vi "Start Counter.vi"(8 "error in (no error)":errorcluster, 10 "ligne index":i32, 11 "Hardware Resources in":T1={"AI"={"task name"="", "task_ref"="", "physical channels"="Dev1/ai0:7", "channels config"={"input terminal configuration"=0, "minimum value"=-5.0, "maximum value"=5.0}, "rate"=1000.0}, "conversions"={"ai0"={"a"=0.0, "b"=0.0}, "ai1"={"a"=0.0, "b"=0.0}, "ai2"={"a"=0.0, "b"=0.0}, "ai3"={"a"=0.0, "b"=0.0}, "ai4"={"a"=0.0, "b"=0.0}}, "compteur 0"={"task name"="CTR", "task_ref"="", "ctr"="Dev1/ctr0:3", "coeff"=4000.0}, "compteur 1"={"task name"="CTR1", "task_ref"="", "ctr"="Dev1/ctr1", "coeff"=4000.0}, "compteur 2"={"task name"="CTR2", "task_ref"="", "ctr"="Dev1/ctr2", "coeff"=4000.0}, "compteur 3"={"task name"="CTR3", "task_ref"="", "ctr"="Dev1/ctr3", "coeff"=4000.0}} {"compteur 3"."coeff" format="%0.2f"; "compteur 2"."coeff" format="%0.2f"; "compteur 1"."coeff" format="%0.2f"; "compteur 0"."coeff" format="%0.2f"; "AI"."rate" format="%0.2f"; "AI"."channels config"."input terminal configuration" items=["Default"=-1, "RSE"=10083, "NRSE"=10078, "Differential"=10106, "Pseudodifferential"=12529]}) -> (0 "error out":errorcluster)   [LabVIEW 2014, in "PLS Acquisition.lvlib"]
doc: "Stops the acquisition."
uses:
  PLS Acquisition.lvlib
  Hardware Configuration.ctl
  Settings/conversion.ctl
  Settings/PLS Settings.lvlib
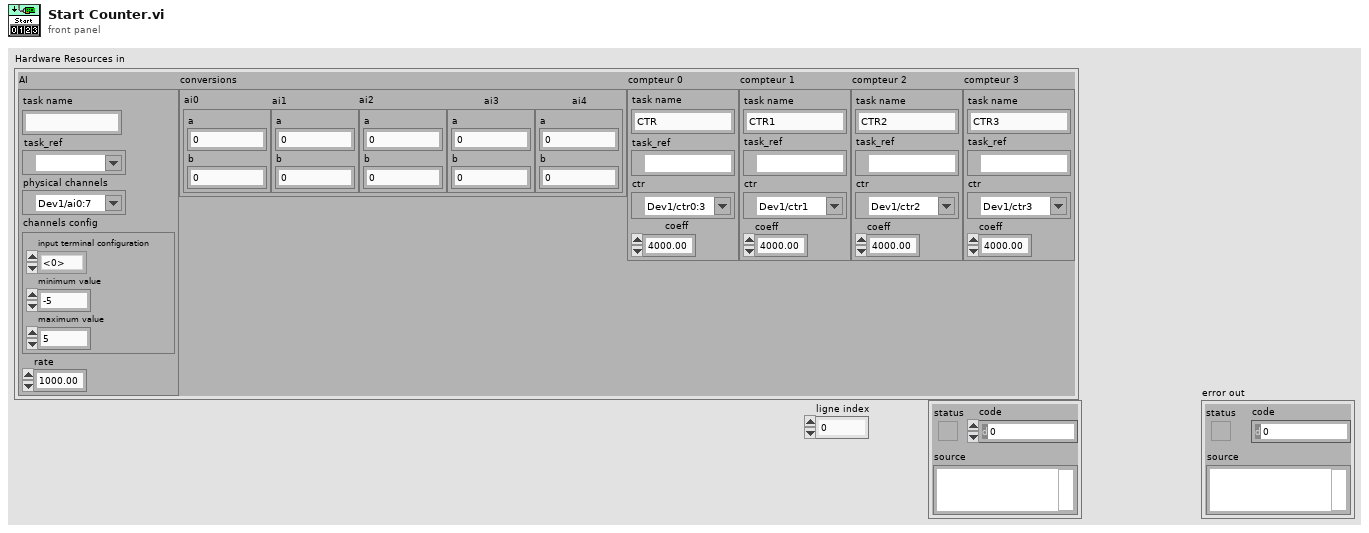
[diagram p1: front panel]
types:
  T1 = typedef "PLS Acquisition.lvlib/Hardware Configuration.ctl" = cluster{"AI":cluster{"task name":string, "task_ref":refnum<k21>, "physical channels":tag, "channels config":cluster{"input terminal configuration":i32, "minimum value":dbl, "maximum value":dbl}, "rate":dbl}, "conversions":cluster{"ai0":T2, "ai1":T2, "ai2":T2, "ai3":T2, "ai4":T2}, "compteur 0":cluster{"task name":string, "task_ref":refnum<k21>, "ctr":tag, "coeff":dbl}, "compteur 1":cluster{"task name":string, "task_ref":refnum<k21>, "ctr":tag, "coeff":dbl}, "compteur 2":cluster{"task name":string, "task_ref":refnum<k21>, "ctr":tag, "coeff":dbl}, "compteur 3":cluster{"task name":string, "task_ref":refnum<k21>, "ctr":tag, "coeff":dbl}}
  T2 = typedef "PLS Settings.lvlib/conversion.ctl" = cluster{"a":dbl, "b":dbl}
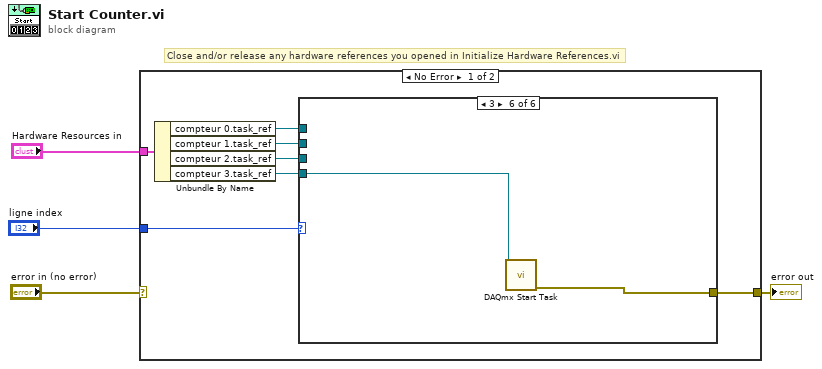
[diagram p0: block diagram]
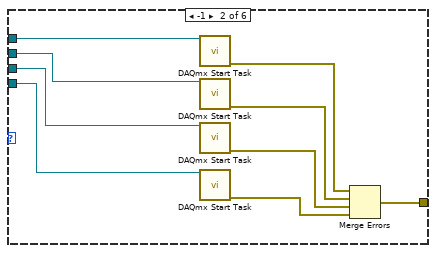
[diagram p3: hidden frame]
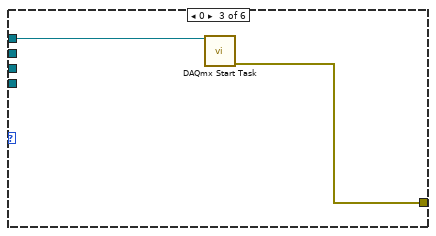
[diagram p4: hidden frame]
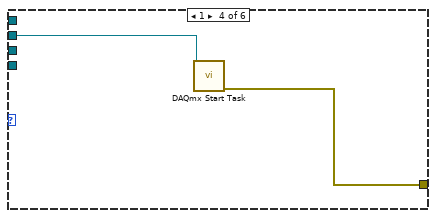
[diagram p5: hidden frame]
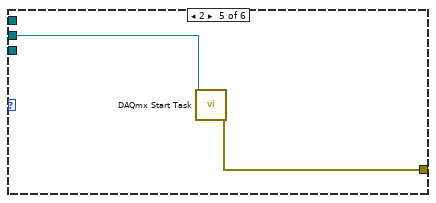
[diagram p6: hidden frame]
diagram:
  # "Close and/or release any hardware references you opened in Initialize Hardware References.vi"
  n1 = case shown="No Error" "error in (no error)" {
    selector: "error in (no error)" -> [_ w29]
    tunnel: [w11 w29] -> w3
    tunnel: "Hardware Resources in" -> [w10 _]
    tunnel: "ligne index" -> [w5 _]
    frame No Error {
      n2 = Unbundle By Name(w10) -> ("compteur 0.task_ref"=w9:refnum<k21>, "compteur 1.task_ref"=w8:refnum<k21>, "compteur 2.task_ref"=w7:refnum<k21>, "compteur 3.task_ref"=w6:refnum<k21>)
      n3 = case shown="3" w5 {
        tunnel: [_ w20 w21 w23 w25 w27] -> w11
        tunnel: w9 -> [_ w19 w22 _ _ _]
        tunnel: w8 -> [_ w15 _ w24 _ _]
        tunnel: w7 -> [_ w17 _ _ w26 _]
        tunnel: w6 -> [_ w16 _ _ _ w28]
        frame Default {
        }
        frame -1 {
          n4 = call <vilib>:"DAQmx Start Task.vi"("task/channels in"=w19) -> ("error out"=w18:errorcluster)  [unwired: 13 in, 1 out]
          n5 = call <vilib>:"DAQmx Start Task.vi"("task/channels in"=w15) -> ("error out"=w14:errorcluster)  [unwired: 13 in, 1 out]
          n6 = call <vilib>:"DAQmx Start Task.vi"("task/channels in"=w17) -> ("error out"=w13:errorcluster)  [unwired: 13 in, 1 out]
          n7 = call <vilib>:"DAQmx Start Task.vi"("task/channels in"=w16) -> ("error out"=w12:errorcluster)  [unwired: 13 in, 1 out]
          n8 = Merge Errors(w18, w14, w13, w12) -> (w20:errorcluster)
        }
        frame 0 {
          n9 = call <vilib>:"DAQmx Start Task.vi"("task/channels in"=w22) -> ("error out"=w21:errorcluster)  [unwired: 13 in, 1 out]
        }
        frame 1 {
          n10 = call <vilib>:"DAQmx Start Task.vi"("task/channels in"=w24) -> ("error out"=w23:errorcluster)  [unwired: 13 in, 1 out]
        }
        frame 2 {
          n11 = call <vilib>:"DAQmx Start Task.vi"("task/channels in"=w26) -> ("error out"=w25:errorcluster)  [unwired: 13 in, 1 out]
        }
        frame 3 {
          n12 = call <vilib>:"DAQmx Start Task.vi"("task/channels in"=w28) -> ("error out"=w27:errorcluster)  [unwired: 13 in, 1 out]
        }
      }
    }
    frame Error {
    }
  }
  "error out" <- w3
